vi "Get Payload.vi"(7 "Msg":refnum<class "Msg.lvclass">) -> (3 "Payload":T1)   [LabVIEW 2020, in "_Template.lvlib" / "{{Msg}}.lvlib" / "Msg.lvclass"]
uses:
  Msg.lvclass
  Msg.lvclass/Msg.ctl
  Payload.ctl
  {{Msg}}.lvlib
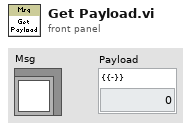
[diagram p1: front panel]
types:
  T1 = typedef "_Template.lvlib/{{Msg}}.lvlib/Payload.ctl" = cluster{"{{-}}":u8}
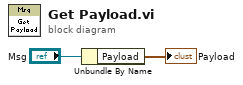
[diagram p0: block diagram]
diagram:
  n1 = Unbundle By Name("Msg") -> ("Payload"=→"Payload":T1)
